vi "Read Payload.vi"(8 "error in":errorcluster, 11 "CoreOOB_Tx in":refnum<class "CIFTemplateCoreOOB_Tx.lvclass">) -> (0 "error out":errorcluster, 2 "data":T1 {"Status"."Custom 8" format="%#_13g"}, 3 "CoreOOB_Tx out":refnum<class "CIFTemplateCoreOOB_Tx.lvclass">)   [LabVIEW 2021, in "CIFTemplateCoreOOB_Tx.lvclass"]
uses:
  CIFTemplateCoreOOB_Tx.lvclass
  D:/dev/CIF-Core-LabVIEW/src/CIFUtilities/CifOutOfBand/CIFOutOfBand.lvclass
  Typedef/Template Payload.ctl
  CIFTemplateCommon/Typedef/Plugin Status.ctl
  CIFTemplateCommon/Typedef/Plugin State.ctl
  CIFTemplateCommon/Typedef/Simple Error.ctl
  CIFUtilities/CifOutOfBand/CIFOutOfBand.lvclass/CIFOutOfBand.ctl
  CIFTemplateCoreOOB_Tx.lvclass/CIFTemplateCoreOOB_Tx.ctl
  CIFUtilities/CifOutOfBand/CIFOutOfBand.lvclass
  CIFTemplateCommon/CIFTemplateCommon.lvlib
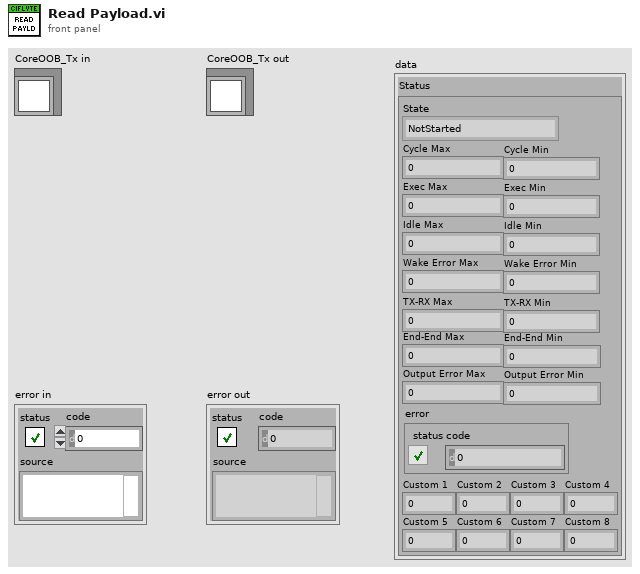
[diagram p1: front panel]
types:
  T1 = typedef "CIFTemplateCoreOOB_Tx.lvclass/Template Payload.ctl" = cluster{"Status":T2}
  T2 = typedef "CIFTemplateCommon.lvlib/Plugin Status.ctl" = cluster{"State":T3, "Cycle Max":i32, "Cycle Min":i32, "Exec Max":i32, "Exec Min":i32, "Idle Max":i32, "Idle Min":i32, "Wake Error Max":i32, "Wake Error Min":i32, "TX-RX Max":i32, "TX-RX Min":i32, "End-End Max":i32, "End-End Min":i32, "Output Error Max":i32, "Output Error Min":i32, "error":T4, "Custom 1":u64, "Custom 2":u64, "Custom 3":u64, "Custom 4":u64, "Custom 5":dbl, "Custom 6":dbl, "Custom 7":dbl, "Custom 8":dbl}
  T3 = typedef "CIFTemplateCommon.lvlib/Plugin State.ctl" = enum32{"NotStarted", "Initialized", "Ready", "Running", "Shutdown"}
  T4 = typedef "CIFTemplateCommon.lvlib/Simple Error.ctl" = cluster{"status":bool, "code":i32}
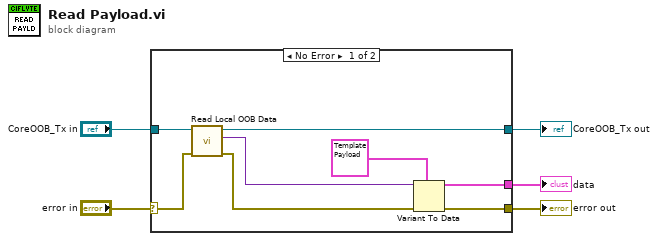
[diagram p0: block diagram]
diagram:
  n1 = case shown="No Error" "error in" {
    selector: "error in" -> [w12 w15]
    tunnel: [w11 w15] -> w5
    tunnel: [w8 w14] -> w4
    tunnel: "CoreOOB_Tx in" -> [w13 w14]
    tunnel: [w7 _] -> w1
    frame No Error {
      n2 = call "Read Local OOB Data.vi"("error in"=w12, "OOB in"=w13) -> ("error out"=w10:errorcluster, "Local OOB Data"=w9:variant, "OOB out"=w8:refnum<class "CIFTemplateCoreOOB_Tx.lvclass">)  [unwired: 7 in]
      n3 = Variant To Data(error in=w10, type=T1 {"Status"={"State"=enum."NotStarted", "Cycle Max"=0, "Cycle Min"=0, "Exec Max"=0, "Exec Min"=0, "Idle Max"=0, "Idle Min"=0, "Wake Error Max"=0, "Wake Error Min"=0, "TX-RX Max"=0, "TX-RX Min"=0, "End-End Max"=0, "End-End Min"=0, "Output Error Max"=0, "Output Error Min"=0, "error"={"status"=FALSE, "code"=0}, "Custom 1"=0, "Custom 2"=0, "Custom 3"=0, "Custom 4"=0, "Custom 5"=0.0, "Custom 6"=0.0, "Custom 7"=0.0, "Custom 8"=0.0}} ("Template Payload"), Variant=w9) -> (data=w7:T1, error out=w11:errorcluster)
    }
    frame Error {
    }
  }
  "error out" <- w5
  "CoreOOB_Tx out" <- w4
  "data" <- w1
